vi "ZLIB Extract All Files To Dir__ogtk.vi"(6 "password (none)":string, 8 "error in (no error)":errorcluster, 10 "root directory (archive name without ending)":path, 11 "archive name (file dialog)":path) -> (0 "error out":errorcluster, 2 "root directory out":path, 3 "archive name out":path)   [LabVIEW 2014]
doc: "This function accepts a zip archive file name and extracts all its files into the directory specified in the root directory input. If no archive file input is specified a file dialog prompts the user to select an archive file. If no root directory is specified a directory with the same name minus file extension and in the same location as the archive is created. Files in archives can have relative paths, which this function will respect, creating subdirectories as needed in the root directory.\n\npassword specifies a necessary password if the archive is encrypted. Leave this parameter empty if the password is not encrypted."
uses:
  <userlib>/_OpenG.lib/file/file.llb/Valid Path - Traditional__ogtk.vi
  <userlib>/_OpenG.lib/file/file.llb/Convert File Extension (Path)__ogtk.vi
  <userlib>/_OpenG.lib/lvzip/lvzip.llb/ZLIB Open Unzip Archive__ogtk.vi
panel:
  # "ZLIB Extract All Files To Dir.vi\n\nThis function accepts a zip archive file name and extracts all its files into a directory\n\nPlease visit http://www.OpenG.org to learn about the\nOpen Source LabVIEW software movement.\n\nNOTICE -- YOU MUST LEAVE THIS NOTICE IN PLACE.  PER THE TERMS OF THE LICENSE BELOW, YOU MAY SUBLICENSE THIS SOFTWARE \nIN ANY WAY THAT DOES NOT CONFLICT WITH THIS LICENSE.\n\n### BSD License (http://www.opensource.org/licenses/bsd-license.php) Begin ###\n \nCopyright (C) 2002 Rolf Kalbermatter rolf.kalbermatter@citeng.com\nCopyright (C) 2002 Jim Kring jim@jimkring.com\n\nAll rights reserved.\n\nRedistribution and use in source and binary forms, with or without modification, are permitted provided that the following conditions are met:\n\n    * Redistributions of source code must retain the above copyright notice, this list of conditions and the following disclaimer.\n    * Redistributions in binary form must reproduce the above copyright notice, this list of conditions and the following disclaimer in the \n       documentation and/or other materials provided with the distribution.\n    * Neither the name of SciWare, James Kring, Inc., nor the names of its contributors may be used to endorse or promote products derived \n       from this software without specific prior written permission.\n\nTHIS SOFTWARE IS PROVIDED BY THE COPYRIGHT HOLDERS AND CONTRIBUTORS \"AS IS\" AND ANY EXPRESS OR IMPLIED WARRANTIES, \nINCLUDING, BUT NOT LIMITED TO, THE IMPLIED WARRANTIES OF MERCHANTABILITY AND FITNESS FOR A PARTICULAR PURPOSE ARE \nDISCLAIMED. IN NO EVENT SHALL THE COPYRIGHT OWNER OR CONTRIBUTORS BE LIABLE FOR ANY DIRECT, INDIRECT, INCIDENTAL,\n SPECIAL, EXEMPLARY, OR CONSEQUENTIAL DAMAGES (INCLUDING, BUT NOT LIMITED TO, PROCUREMENT OF SUBSTITUTE GOODS OR \nSERVICES; LOSS OF USE, DATA, OR PROFITS; OR BUSINESS INTERRUPTION) HOWEVER CAUSED AND ON ANY THEORY OF LIABILITY, \nWHETHER IN CONTRACT, STRICT LIABILITY, OR TORT (INCLUDING NEGLIGENCE OR OTHERWISE) ARISING IN ANY WAY OUT OF THE USE \nOF THIS SOFTWARE, EVEN IF ADVISED OF THE POSSIBILITY OF SUCH DAMAGE.\n\n### BSD License End ###"
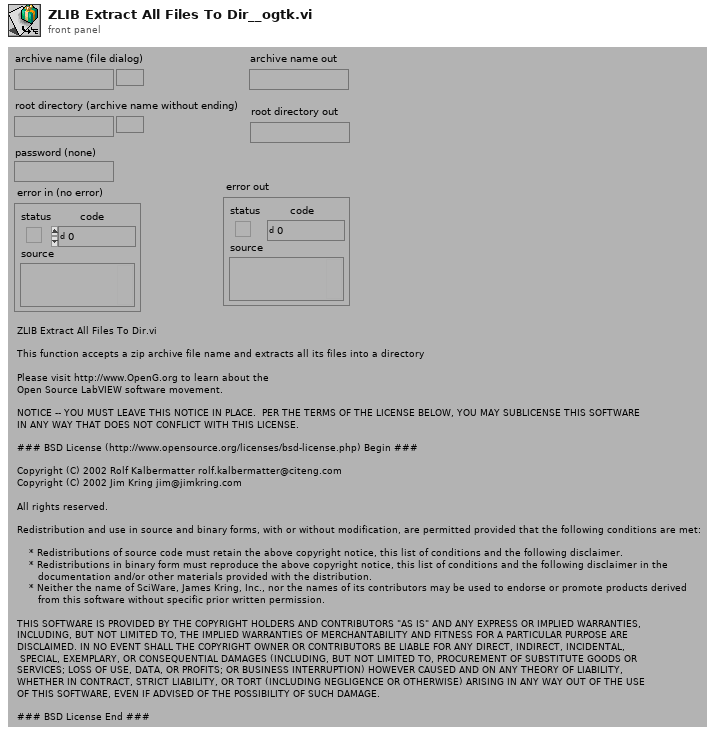
[diagram p1: front panel]
types:
  T1 = enum32{"existing file", "new file", "new or existing file", "existing dir", "new dir", "new or existing dir", "existing file (use LLBs)", "new file (use LLBs)", "new or existing file (use LLBs)", "new or existing file or directory (use LLBs)", "existing dir (use LLBs)", "new dir (use LLBs)", "new or existing dir (use LLBs)", "existing file or dir", "new file or dir", "new or existing file or dir", "existing file or dir (use LLBs)", "new file or dir (use LLBs)"}
  T2 = typedef "ZLIB Unzip Handle__ogtk.ctl" = refnum<k1>
  T3 = typedef "ZLIB File Info__ogtk.ctl" = cluster{"version":u32, "version needed":u32, "encrypted":bool, "flag":u32, "compression":i32, "dos date":u32, "crc":u32, "compressed size":u32, "uncompressed size":u32, "extra info":string, "file comment":string, "disk num start":u32, "internal fa":u32, "external fa":u32, "file timestamp":u32}
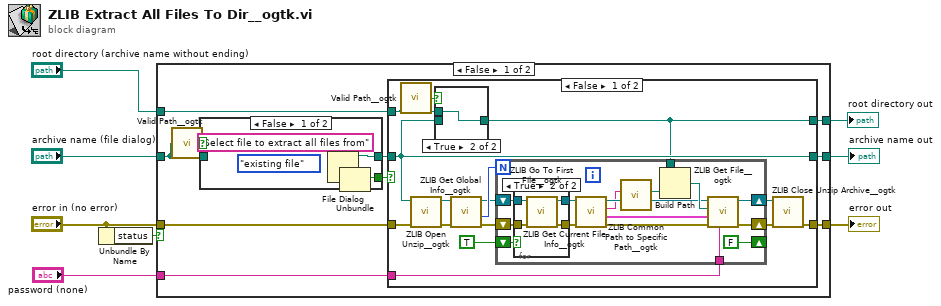
[diagram p0: block diagram]
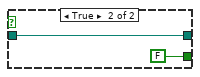
[diagram p2: hidden frame]
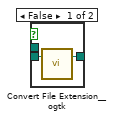
[diagram p3: hidden frame]
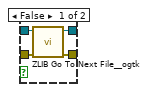
[diagram p4: hidden frame]
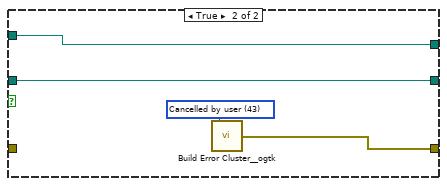
[diagram p5: hidden frame]
diagram:
  n1 = Unbundle By Name("error in (no error)") -> ("status"=w6:bool)
  n2 = case shown="False" w6 {
    tunnel: "archive name (file dialog)" -> [w16 w72]
    tunnel: "error in (no error)" -> [w14 w73]
    tunnel: [w13 w73] -> w5
    tunnel: [w12 w72] -> w4
    tunnel: [w11 w71] -> w3
    tunnel: "root directory (archive name without ending)" -> [w10 w71]
    tunnel: "password (none)" -> [w9 _]
    frame False {
      n3 = call-poly <userlib>:"Valid Path__ogtk.vi"("path"=w16) -> ("valid"=w15:bool)
      n4 = case shown="False" w15 {
        tunnel: [w21 w24] -> w18
        tunnel: [w20 FALSE ("cancelled")] -> w17
        tunnel: w16 -> [_ w24]
        frame False {
          (unwired) T1."existing file" ("select mode (2)")
          n5 = File Dialog(7:"Select file to extract all files from" ("prompt")) -> (0:w19:errorcluster, 1:w20:bool, 3:w21:path)  [unwired: 6 in, 1 out]
          n6 = Unbundle(w19) -> ()  [unwired: 3 out]
        }
        frame True {
        }
      }
      n7 = case shown="False" w17 {
        tunnel: w18 -> [w33 w68]
        tunnel: [w37 w69] -> w13
        tunnel: w10 -> [w36 w67]
        tunnel: w14 -> [w34 _]
        tunnel: [w33 w68] -> w12
        tunnel: [w32 w67] -> w11
        tunnel: w9 -> [w31 _]
        frame False {
          n8 = call-poly <userlib>:"Valid Path__ogtk.vi"("path"=w36) -> ("valid"=w35:bool)
          n9 = call-poly <userlib>:"ZLIB Open Unzip__ogtk.vi"("error in (no error)"=w34, "archive name"=w33) -> ("error out"=w30:errorcluster, "unzip Refnum"=w28:T2)  [unwired: 4 in]
          n10 = case shown="True" w35 {
            tunnel: w33 -> [w41 _]
            tunnel: [w40 w42] -> w32
            tunnel: w36 -> [_ w42]
            frame False {
              n11 = call-poly <userlib>:"Convert File Extension__ogtk.vi"("file name"=w41) -> ("new filename"=w40:path)  [unwired: 1 in, 1 out]
            }
            frame True {
            }
          }
          n12 = call <userlib>:"ZLIB Get Global Info__ogtk.vi"("error in (no error)"=w30, "unzip Refnum"=w28) -> ("error out"=w26:errorcluster, "nEntry"=w29:u32, "unzip Refnum out"=w27:T2)  [unwired: 2 in, 1 out]
          n13 = for {
            N: w29 -> [_]
            shift-right: [w58] -> w39
            shift-left: w27 -> [w51]
            shift-right: [w57] -> w38
            shift-left: w26 -> [w52]
            tunnel: w32 -> [w56]
            tunnel: w31 -> [w53]
            shift-right: [FALSE] -> _
            shift-left: TRUE -> [w48]
            n14 = case shown="True" w48 {
              tunnel: w51 -> [w61 w66]
              tunnel: w52 -> [w62 w65]
              tunnel: [w60 w64] -> w50
              tunnel: [w59 w63] -> w49
              frame False {
                n15 = call <userlib>:"ZLIB Go To Next File__ogtk.vi"("error in (no error)"=w62, "unzip Refnum"=w61) -> ("error out"=w59:errorcluster, "unzip Refnum out"=w60:T2)  [unwired: 4 in]
              }
              frame True {
                n16 = call <userlib>:"ZLIB Go To First File__ogtk.vi"("error in (no error)"=w65, "unzip Refnum"=w66) -> ("error out"=w63:errorcluster, "unzip Refnum out"=w64:T2)  [unwired: 4 in]
              }
            }
            n17 = call <userlib>:"ZLIB Get Current File Info__ogtk.vi"("error in (no error)"=w49, "unzip Refnum"=w50) -> ("error out"=w45:errorcluster, "file info"=w43:T3, "name"=w44:string, "unzip Refnum out"=w46:T2)  [unwired: 6 in]
            n18 = call <userlib>:"ZLIB Common Path to Specific Path__ogtk.vi"("common path"=w44) -> ("specific path"=w54:path)  [unwired: 10 in]
            n19 = Build Path(base path=w56, name or relative path=w54) -> (appended path=w55:path)
            n20 = call <userlib>:"ZLIB Get File__ogtk.vi"("password (none)"=w53, "error in (no error)"=w45, "file info"=w43, "target path"=w55, "unzip Refnum"=w46) -> ("error out"=w57:errorcluster, "unzip Refnum out"=w58:T2)  [unwired: 3 in]
          }
          n21 = call <userlib>:"ZLIB Close Unzip Archive__ogtk.vi"("error in (no error)"=w38, "unzip Refnum"=w39) -> ("error out"=w37:errorcluster)  [unwired: 5 in]
        }
        frame True {
          w70 = 43 items=["No error", "Argument error", "Memory is full", "Out of zone", "End of file", "File already open", "Generic file I/O error", "File not found", "File permission error", "Disk is full", "Duplicate path", "Too many files open", "System feature not enabled", "Resource file not found", "Cannot add resource", "Resource not found", "Image not found", "Image memory error", "Pen does not exist", "Config type invalid", "Config token not found", "Config parse error", "Config memory error", "Bad external code format", "Bad external code offset", "External code not present", "Null window", "Destroy window error", "Null menu", "Print aborted", "Bad print record", "Print driver error", "Windows error during printing", "Memory error during printing", "Print dialog error", "Generic print error", "Invalid device refnum", "Device not found", "Device parameter error", "Device unit error", "Cannot open device", "Device call aborted", "Generic error", "Cancelled by user", "Object ID too low", "Object ID too high", "Object not in heap", "Unknown heap", "Unknown object (invalid DefProc)", "Unknown object (DefProc not in table)", "Message out of range", "Invalid (null) method", "Unknown message", "Manager call not supported", "Bad address", "Network operation in progress", "Network operation timed out", "Connection is busy", "Network attribute not supported", "Network error", "Address in use", "System out of memory", "Connection aborted", "Connection refused", "Not connected", "Already connected", "Connection closed", "Initialization error (interapplication manager)", "Bad occurrence", "Wait on unbound occurrence handler", "Occurrence queue overflow", "Datalog type conflict", "Unused", "Unrecognized type (interapplication manager)", "Memory corrupt", "Failed to make temporary DLL", "Old CIN version", "Drag socket not found", "Failed to load drop-object", "Failed to register OLE object", "Failed to release OLE object", "Format specifier type mismatch", "Unknown format specifier", "Too few format specifiers", "Too many format specifiers", "Scan failed", "Newer CIN version", "Error converting to variant", "Runtime menu error", "Password tampered", "Variant attribute not found", "Incompatible variant data type", "Event data is not available", "Event Store is not present", "Occurrence is not found", "Event Queue is not created", "Event info is not available", "Refnum passed is NULL", "Error retrieving Class GUID", "Error retrieving CoClass GUID", "Error retrieving TypeLib GUID.", "Bad built application magic bytes.", "Specific driver is different from the specific driver associated with the Logical Name.", "There is no session opened to the class driver.", "Max Error", "MAX - Error with config objects", "MAX - Error loading configuration", "MAX - Group not supported"]
          n22 = call <userlib>:"Build Error Cluster__ogtk.vi"("code"=w70) -> ("error out"=w69:errorcluster)  [unwired: 1 in]
        }
      }
    }
    frame True {
    }
  }
  "error out" <- w5
  "archive name out" <- w4
  "root directory out" <- w3
